vi "SetupAnalog.vi"() -> ()   [LabVIEW 2009]
uses:
  AnalogSettings.ctt
panel:
  in  "OK Button":bool
  in  "Cancel Button":bool
  in  "Analog Settings":T1={"PCI 671x Device Number"=1, "Samples per Unit"=10}
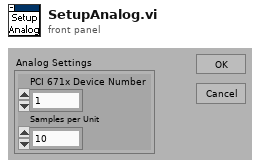
[diagram p1: front panel]
types:
  T1 = typedef "AnalogSettings.ctt" = cluster{"PCI 671x Device Number":u32, "Samples per Unit":u32}
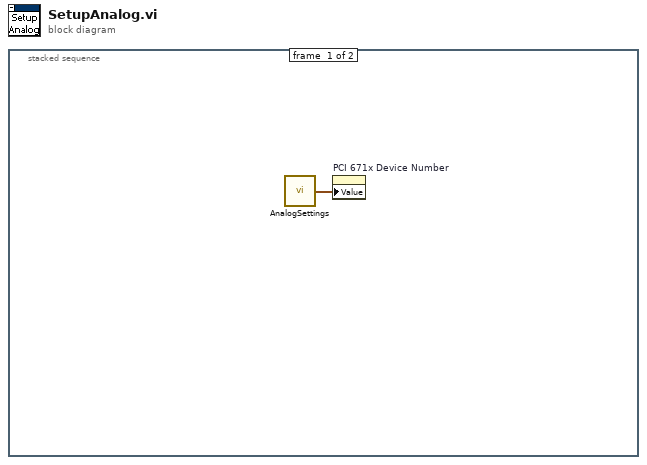
[diagram p0: block diagram]
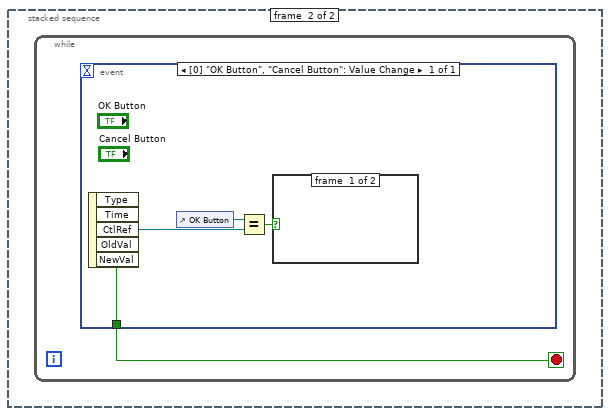
[diagram p2: hidden frame]
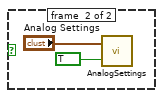
[diagram p3: hidden frame]
diagram:
  n1 = stacked-sequence {
    frame #0 {
      n2 = call "AnalogSettings.vi"() -> ("Analog Settings (output)"=w1:T1)  [unwired: 2 in]
      n3 = property on="PCI 671x Device Number" class="Clust (strict)"("Value"=w1) -> ()  [unwired: 2 in, 2 out]
    }
    frame #1 {
      n4 = while {
        stop <- w2 stop-if-true
        n5 = event shown="[0] \"OK Button\", \"Cancel Button\": Value Change" {
          selector: _ -> [_]
          dyn-events: _ -> [_]
          timeout: _ -> [_]
          tunnel: [w5] -> w2
          event [0] "OK Button", "Cancel Button": Value Change {
            n6 = event-data() -> ("CtlRef"=w6:refnum<vi>, "NewVal"=w5:bool)  [unwired: 1 in, 3 out]
            n7 = control-ref of="OK Button"() -> (w4:refnum<vi>)
            n8 = Equal?(x=w4, y=w6) -> (x = y?=w3:bool)
            n9 = case shown="True" w3 {
              frame #0 {
              }
              frame #1 {
                n10 = call "AnalogSettings.vi"("Get/Set"=TRUE, "Analog Settings (input)"="Analog Settings") -> ()  [unwired: 1 out]
              }
            }
          }
        }
      }
    }
  }
